vi "Correction.vi"() -> ()   [LabVIEW 2016]
doc: "This example shows how to use the Edge Tool in NI Vision. The Edge Tool finds edges (or sharp transitions in the pixels values) along a given line or ROI profile. The Edge Tool is a precursor function to many of the gauging and inspection tasks. For example, the location of the edges found along a line profile across an object can interpreted as the boundaries of the object whose dimensions have to be measured for a gauging application or the presence of a crack in the surface of an object for an inspection application."
uses:
  <vilib>/vision/Process.llb/Background Estimation Options.ctl
  <vilib>/vision/Process.llb/Surface Fit Options.ctl
  <vilib>/vision/NI_Vision_Development_Module.lvlib
panel:
  in  "Tab":enum32{"Src", "FlatFied", "Corrected"}(tab)
  out "Src":T1(plugin-control)
  out "FField":T1(plugin-control)
  out "Img":T1(plugin-control)
  in  "Surface Fit Options":T2={"Model"=0, "Sampling Grid Size"={"SizeX"=100, "SizeY"=100}, "Polynomial Degree"=2} {"Sampling Grid Size"."SizeY" min=3 step=1; "Sampling Grid Size"."SizeX" min=3 step=1; "Model" items=["Polynomial"]}
  in  "Background Estimation Options":T3={"Estimate Background?"=FALSE, "Method"=0, "Polynomial Degree"=2, "Window Size (32x32)"={"SizeX"=32, "SizeY"=32}, "Niblack Deviation Factor (0.2)"=0.2} {"Niblack Deviation Factor (0.2)" min=0.0 max=1.0 format="%.2f"; "Window Size (32x32)"."SizeY" min=3 step=1; "Window Size (32x32)"."SizeX" min=3 step=1; "Method" items=["Polynomial", "Background Correction", "NiBlack"]}
  in  "Method":T4(ring)
  in  "Stop":bool
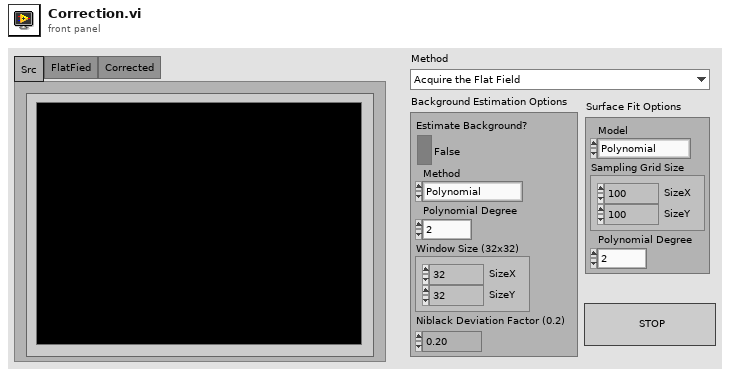
[diagram p1: front panel]
types:
  T1 = typedef "IMAQ Image.ctl" = refnum<image>
  T2 = typedef "Surface Fit Options.ctl" = cluster{"Model":i32, "Sampling Grid Size":cluster{"SizeX":i32, "SizeY":i32}, "Polynomial Degree":i32}
  T3 = typedef "Background Estimation Options.ctl" = cluster{"Estimate Background?":bool, "Method":i32, "Polynomial Degree":i32, "Window Size (32x32)":cluster{"SizeX":i32, "SizeY":i32}, "Niblack Deviation Factor (0.2)":dbl}
  T4 = enum16{"Acquire the Flat Field", "Estimate the Flat Field"}
  T5 = cluster{"Method":enum16{"Acquire the Flat Field", "Estimate the Flat Field"}, "Surface Fit Options":T2, "Background Estimation Options":T3}
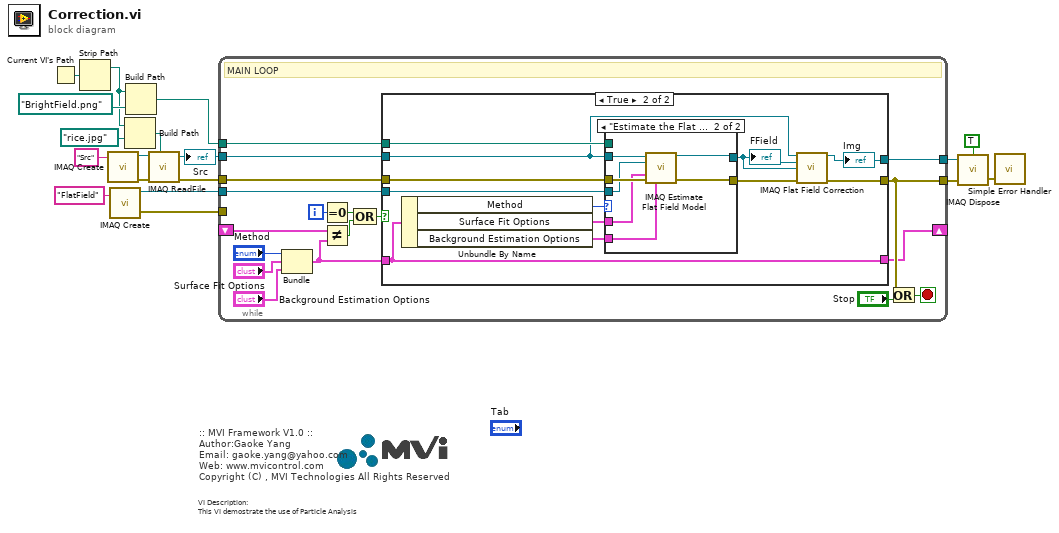
[diagram p0: block diagram]
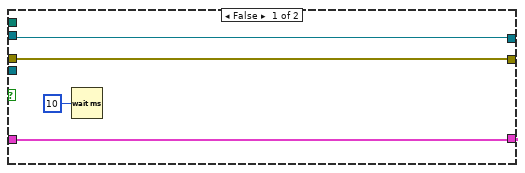
[diagram p2: hidden frame]
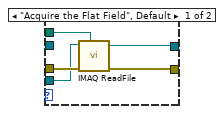
[diagram p3: hidden frame]
diagram:
  # "VI Description:\nThis VI demostrate the use of Particle Analysis"
  # ":: MVI Framework V1.0 ::\nAuthor:Gaoke Yang\nEmail: gaoke.yang@yahoo.com\nWeb: www.mvicontrol.com\nCopyright (C) , MVI Technologies All Rights Reserved"
  n1 = Current VI's Path() -> (path=w9:path)
  n2 = Strip Path(path=w9) -> (stripped path=w3:path)  [unwired: 1 out]
  n3 = call "IMAQ Create"("Image Name"="Src") -> ("New Image"=w17:T1, "error out"=w16:errorcluster)  [unwired: 4 in]
  n4 = call "IMAQ Create"("Image Name"="FlatField") -> ("New Image"=w6:T1, "error out"=w5:errorcluster)  [unwired: 4 in]
  n5 = Build Path(base path=w3, name or relative path=path "rice.jpg" ("prompt")) -> (appended path=w8:path)
  n6 = Build Path(base path=w3, name or relative path=path "BrightField.png" ("prompt")) -> (appended path=w2:path)
  n7 = call "IMAQ ReadFile"("File Path"=w8, "error in (no error)"=w16, "Image"=w17) -> ("error out"=w11:errorcluster, "Image Out"=w1:T1)  [unwired: 4 in, 3 out]
  "Src" <- w1
  n8 = while "MAIN LOOP" {
    tunnel: w1 -> [w26]
    tunnel: w11 -> [w25]
    tunnel: [w33] -> w15
    tunnel: [w34] -> w14
    shift-right: [w30] -> _
    shift-left: _ -> [w23]
    tunnel: w6 -> [w27]
    tunnel: w5 -> [_]
    tunnel: w2 -> [w21]
    i -> [w32]
    stop <- w35 stop-if-true
    # "MAIN LOOP"
    n9 = Bundle("Method"="Method", "Surface Fit Options"="Surface Fit Options", "Background Estimation Options"="Background Estimation Options") -> (w22:T5)  [unwired: 1 in]
    n10 = Equal To 0?(x=w32) -> (x = 0?=w29:bool)
    n11 = Not Equal?(x=w23, y=w22) -> (x != y?=w28:bool)
    n12 = Compound Arithmetic op=OR(w29, w28) -> (w31:bool)
    n13 = case shown="True" w31 {
      tunnel: w25 -> [w39 w49]
      tunnel: w26 -> [w40 w44]
      tunnel: [w40 w42] -> w34
      tunnel: [w39 w43] -> w33
      tunnel: [w38 w52] -> w30
      tunnel: w22 -> [w38 w52]
      tunnel: w27 -> [_ w48]
      tunnel: w21 -> [_ w50]
      frame False {
        n14 = Wait (ms)(milliseconds to wait=u32 10) -> ()  [unwired: 1 out]
      }
      frame True {
        n15 = Unbundle By Name(w52) -> ("Method"=w51:T4, "Surface Fit Options"=w47:T2, "Background Estimation Options"=w46:T3)
        n16 = case shown="\"Estimate the Flat Field\"" w51 {
          tunnel: w50 -> [w53 _]
          tunnel: w49 -> [w57 w64]
          tunnel: w48 -> [w56 w61]
          tunnel: [w55 w63] -> w45
          tunnel: [w54 w62] -> w41
          tunnel: w44 -> [_ w60]
          tunnel: w47 -> [_ w59]
          tunnel: w46 -> [_ w58]
          frame "Acquire the Flat Field", Default {
            n17 = call "IMAQ ReadFile"("File Path"=w53, "error in (no error)"=w57, "Image"=w56) -> ("error out"=w55:errorcluster, "Image Out"=w54:T1)  [unwired: 4 in, 3 out]
          }
          frame "Estimate the Flat Field" {
            n18 = call "IMAQ Estimate Flat Field Model"("Image Src"=w60, "Image Dst"=w61, "Surface Fit Options"=w59, "error in (no error)"=w64, "Background Estimation Options"=w58) -> ("Flat Field Image Out"=w62:T1, "error out"=w63:errorcluster)  [unwired: 9 in]
          }
        }
        "FField" <- w41
        n19 = call "IMAQ Flat Field Correction"("Image Src"=w44, "Image Dst"=w41, "Flat Field Image"=w41, "error in (no error)"=w45) -> ("Corrected Image"=w42:T1, "error out"=w43:errorcluster)  [unwired: 9 in, 1 out]
        "Img" <- w42
      }
    }
    n20 = Or(x=w33, y="Stop") -> (x .or. y?=w35:bool)
  }
  n21 = call "IMAQ Dispose"("All Images? (No)"=TRUE, "Image"=w14, "error in (no error)"=w15) -> ("error out"=w13:errorcluster)  [unwired: 3 in]
  n22 = call <vilib>:"Simple Error Handler.vi"("error in (no error)"=w13) -> ()  [unwired: 4 in, 5 out]
